vi "题目 2.vi"() -> ()   [LabVIEW 2017]
panel:
  out "和 2":i32
  out "和":i32
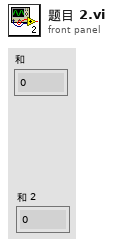
[diagram p1: front panel]
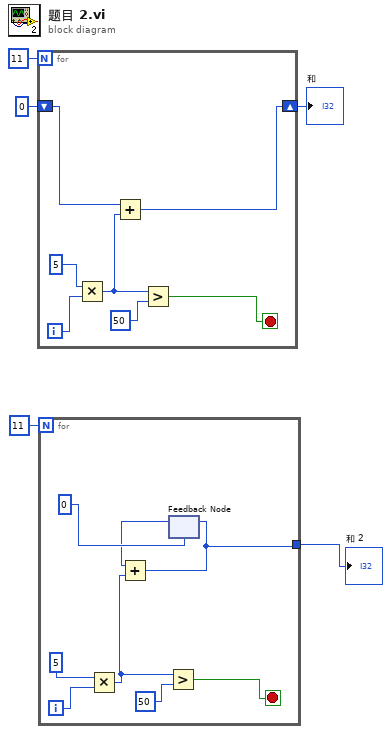
[diagram p0: block diagram]
diagram:
  n1 = for {
    N: 11 -> [_]
    shift-right: [w10] -> w4
    shift-left: 0 -> [w9]
    i -> [w11]
    stop <- w7 stop-if-true
    n2 = Multiply(x=5, y=w11) -> (x*y=w6:i32)
    n3 = Add(x=w9, y=w6) -> (x+y=w10:i32)
    n4 = Greater?(x=w6, y=50) -> (0:w7:bool)
  }
  "和" <- w4
  n5 = for {
    N: 11 -> [_]
    tunnel: [w13] -> w1
    i -> [w19]
    stop <- w14 stop-if-true
    n6 = Multiply(x=5, y=w19) -> (x*y=w17:i32)
    n7 = Greater?(x=w17, y=50) -> (0:w14:bool)
    n8 = feedback #1(0) -> (w15:i32)
    n9 = Add(x=w15, y=w17) -> (x+y=w13:i32)
    n10 = feedback-in #1(w13) -> ()
  }
  "和 2" <- w1
